vi "Chaser_Mk2.vi"   [LabVIEW 2015]
uses:
  <vilib>/Aledyne-TSXperts/Arduino Compatible Compiler for LabVIEW/Code Generator/Arduino APIs/RGB LED Strip/RGB Strip Mode.ctl
  <vilib>/Aledyne-TSXperts/Arduino Compatible Compiler for LabVIEW/Code Generator/Arduino APIs/Serial/Serial Settings.ctl
  <vilib>/Aledyne-TSXperts/Arduino Compatible Compiler for LabVIEW/Arduino Compatible Compiler for LabVIEW.lvlib
types:
  T1 = typedef "Arduino Compatible Compiler for LabVIEW.lvlib/Serial Settings.ctl" = u16
  T2 = typedef "Arduino Compatible Compiler for LabVIEW.lvlib/RGB Strip Mode.ctl" = u16
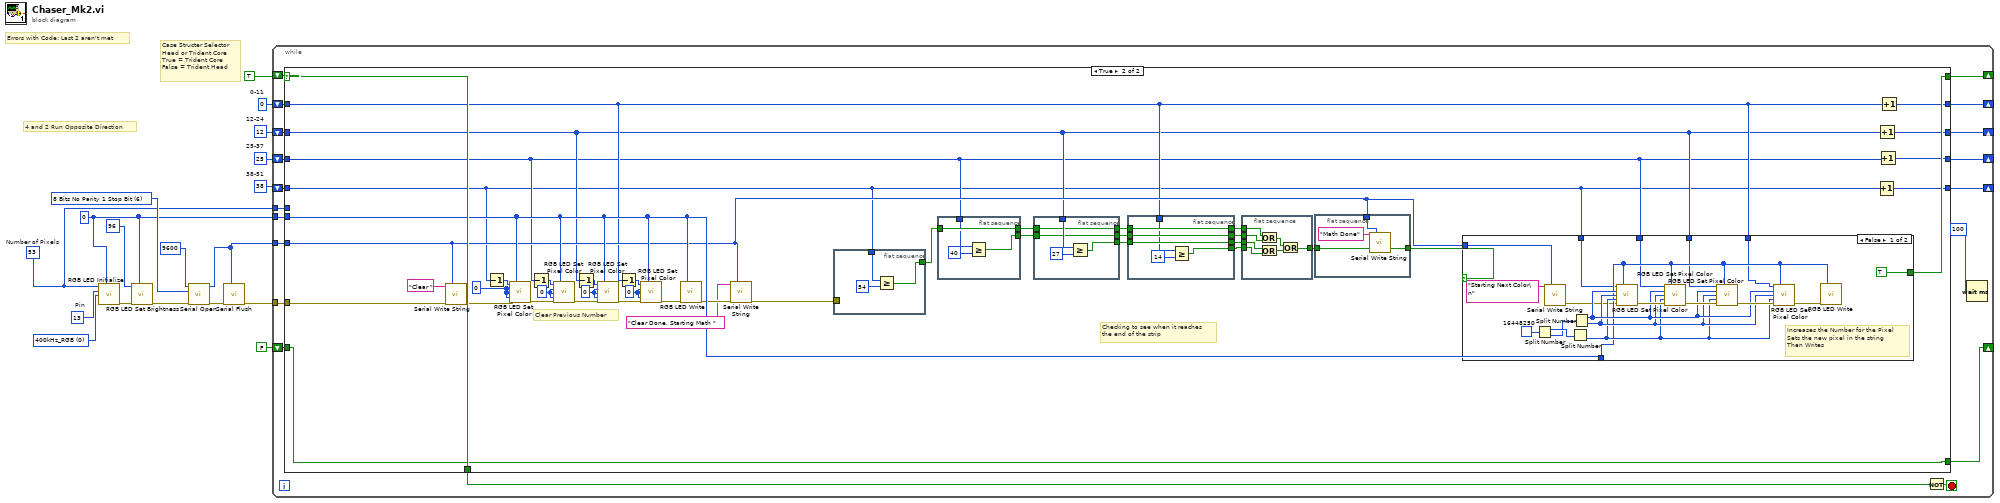
[diagram p0: block diagram]
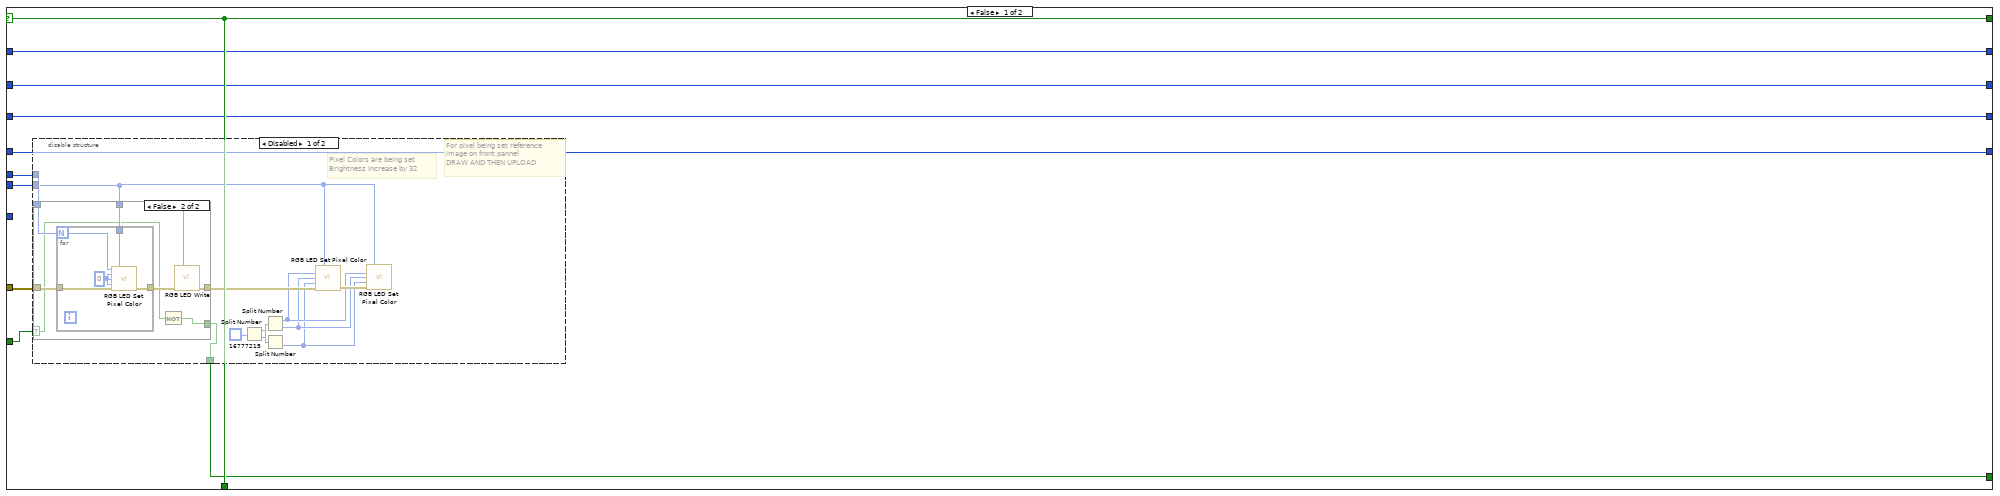
[diagram p2: hidden frame]
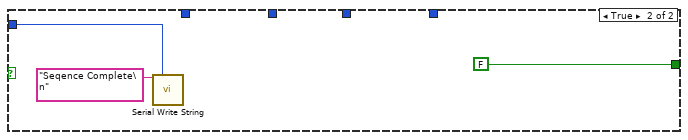
[diagram p5: hidden frame]
diagram:
  w5 = u16 38  # 38-51
  w6 = u16 25  # 25-37
  w7 = u16 12  # 12-24
  w8 = u16 0  # 0-11
  w13 = T1 6 items=["5 Bits No Parity 1 Stop Bit"=0, "6 Bits No Parity 1 Stop Bit"=2, "7 Bits No Parity 1 Stop Bit"=4, "8 Bits No Parity 1 Stop Bit"=6, "5 Bits No Parity 2 Stop Bits"=8, "6 Bits No Parity 2 Stop Bits"=10, "7 Bits No Parity 2 Stop Bits"=12, "8 Bits No Parity 2 Stop Bits"=14, "5 Bits Even Parity 1 Stop Bits"=32, "6 Bits Even Parity 1 Stop Bits"=34, "7 Bits Even Parity 1 Stop Bits"=36, "8 Bits Even Parity 1 Stop Bits"=38, "5 Bits Even Parity 2 Stop Bits"=40, "6 Bits Even Parity 2 Stop Bits"=42, "7 Bits Even Parity 2 Stop Bits"=44, "8 Bits Even Parity 2 Stop Bits"=46, "5 Bits Odd Parity 1 Stop Bits"=48, "6 Bits Odd Parity 1 Stop Bits"=50, "7 Bits Odd Parity 1 Stop Bits"=52, "8 Bits Odd Parity 1 Stop Bits"=54, "5 Bits Odd Parity 2 Stop Bits"=56, "6 Bits Odd Parity 2 Stop Bits"=58, "7 Bits Odd Parity 2 Stop Bits"=60, "8 Bits Odd Parity 2 Stop Bits"=62] ("Serial Settings")
  w17 = T2 0 items=["400kHz_RGB"=0, "400kHz_GRB"=1, "400kHz_BRG"=4, "800kHz_RGB"=2, "800kHz_GRB"=3, "400kHz_BRG"=6] ("Mode")
  w18 = u8 13  # Pin
  w2 = u8 53  # Number of Pixels
  w4 = u8 0 ("Instance")
  # "Errors with Code: Last 2 aren't met"
  # "4 and 2 Run Opposite Direction"
  # "Case Structer Selector\nHead or Trident Core\nTrue = Trident Core\nFalse = Trident Head"
  n1 = call <vilib>:"RGB LED Initialize.vi"("Number of Pixels"=w2, "Instance"=w4, "Pin"=w18, "Mode"=w17) -> ("error out"=w16:errorcluster)  [unwired: 11 in]
  n2 = call <vilib>:"RGB LED Set Brightness.vi"("Brightness"=u8 96, "Instance"=w4, "error in (no error)"=w16) -> ("error out"=w14:errorcluster)  [unwired: 12 in]
  n3 = call <vilib>:"Serial Open.vi"("Speed"=u32 9600, "Serial Settings"=w13, "error in (no error)"=w14) -> ("Instance"=w3:u8, "error out"=w11:errorcluster)  [unwired: 11 in]
  n4 = call <vilib>:"Serial Flush.vi"("Instance"=w3, "error in (no error)"=w11) -> ("error out"=w10:errorcluster)  [unwired: 13 in]
  n5 = while {
    tunnel: w10 -> [w29]
    shift-right: [w36] -> _
    shift-left: TRUE -> [w37]
    shift-right: [w27] -> _
    shift-left: w8 -> [w33]
    shift-right: [w26] -> _
    shift-left: w7 -> [w32]
    shift-right: [w25] -> _
    shift-left: w6 -> [w31]
    shift-right: [w24] -> _
    shift-left: w5 -> [w30]
    tunnel: w4 -> [w28]
    tunnel: w3 -> [w23]
    tunnel: w2 -> [w21]
    shift-right: [w19] -> _
    shift-left: FALSE -> [w20]
    stop <- w35 stop-if-true
    n6 = case shown="True" w37 {
      selector: w37 -> [w47 w98]
      tunnel: [w47 w97] -> w36
      tunnel: [w47 w98] -> w34
      tunnel: w33 -> [w46 w83]
      tunnel: w32 -> [w45 w81]
      tunnel: w31 -> [w44 w78]
      tunnel: w30 -> [w43 w76]
      tunnel: w29 -> [w41 w88]
      tunnel: w28 -> [w38 w96]
      tunnel: [w46 w82] -> w27
      tunnel: [w45 w80] -> w26
      tunnel: [w44 w79] -> w25
      tunnel: [w43 w77] -> w24
      tunnel: w23 -> [_ w89]
      tunnel: w21 -> [w42 _]
      tunnel: w20 -> [w40 w75]
      tunnel: [w39 w75] -> w19
      frame False {
        n7 = disable-structure shown="Disabled" {
          disable-tunnel: w42 -> [w60 _]
          disable-tunnel: w41 -> [w59 _]
          disable-tunnel: w40 -> [w58 _]
          disable-tunnel: [w57 _] -> w39
          disable-tunnel: w38 -> [w48 _]
          frame Disabled {
            # "For pixel being set reference\nimage on front pannel\nDRAW AND THEN UPLOAD"
            # "Pixel Colors are being set\nBrightness Increase by 32"
            n8 = case shown="False" w58 {
              selector: w58 -> [w61 w64]
              tunnel: w60 -> [_ w69]
              tunnel: w59 -> [w62 w68]
              tunnel: w48 -> [_ w66]
              tunnel: [w62 w65] -> w56
              tunnel: [w61 w63] -> w57
              frame True {
              }
              frame False {
                n9 = for {
                  N: w69 -> [w73]
                  tunnel: w68 -> [w74]
                  tunnel: w66 -> [w71]
                  tunnel: [w70] -> w67
                  w72 = u8 0 ("Green")
                  n10 = call <vilib>:"RGB LED Set Pixel Color.vi"("Pixel"=w73, "Instance"=w71, "Red"=w72, "Green"=w72, "Blue"=w72, "error in (no error)"=w74) -> ("error out"=w70:errorcluster)  [unwired: 9 in]
                }
                n11 = Not(x=w64) -> (.not. x?=w63:bool)
                n12 = call <vilib>:"RGB LED Write.vi"("Instance"=w66, "error in (no error)"=w67) -> ("error out"=w65:errorcluster)  [unwired: 13 in]
              }
            }
            n13 = Split Number(x=u32 16777215) -> (hi(x)=w54:u16, lo(x)=w53:u16)
            n14 = Split Number(x=w53) -> (hi(x)=w51:u8, lo(x)=w50:u8)
            n15 = Split Number(x=w54) -> (lo(x)=w49:u8)  [unwired: 1 out]
            n16 = call <vilib>:"RGB LED Set Pixel Color.vi"("Instance"=w48, "Red"=w51, "Green"=w50, "Blue"=w49, "error in (no error)"=w56) -> ("error out"=w52:errorcluster)  [unwired: 10 in]
            n17 = call <vilib>:"RGB LED Set Pixel Color.vi"("Instance"=w48, "Red"=w51, "Green"=w50, "Blue"=w49, "error in (no error)"=w52) -> ()  [unwired: 10 in, 1 out]
          }
          frame Enabled {
          }
        }
      }
      frame True {
        w112 = u8 0 ("Green")
        w113 = u8 0 ("Green")
        w115 = u8 0 ("Green")
        w116 = u8 0 ("Green")
        # "Checking to see when it reaches\nthe end of the strip"
        # "Clear Previous Number"
        n18 = call <vilib>:"Serial Write String.vi"("String"="Clear ", "Instance"=w89, "error in (no error)"=w88) -> ("error out"=w93:errorcluster)  [unwired: 12 in]
        n19 = Decrement(x=w76) -> (x-1=w87:u16)
        n20 = call <vilib>:"RGB LED Set Pixel Color.vi"("Pixel"=w87, "Instance"=w96, "Red"=w116, "Green"=w116, "Blue"=w116, "error in (no error)"=w93) -> ("error out"=w114:errorcluster)  [unwired: 9 in]
        n21 = Decrement(x=w78) -> (x-1=w86:u16)
        n22 = call <vilib>:"RGB LED Set Pixel Color.vi"("Pixel"=w86, "Instance"=w96, "Red"=w115, "Green"=w115, "Blue"=w115, "error in (no error)"=w114) -> ("error out"=w110:errorcluster)  [unwired: 9 in]
        n23 = Decrement(x=w81) -> (x-1=w85:u16)
        n24 = call <vilib>:"RGB LED Set Pixel Color.vi"("Pixel"=w85, "Instance"=w96, "Red"=w113, "Green"=w113, "Blue"=w113, "error in (no error)"=w110) -> ("error out"=w111:errorcluster)  [unwired: 9 in]
        n25 = Decrement(x=w83) -> (x-1=w84:u16)
        n26 = call <vilib>:"RGB LED Set Pixel Color.vi"("Pixel"=w84, "Instance"=w96, "Red"=w112, "Green"=w112, "Blue"=w112, "error in (no error)"=w111) -> ("error out"=w109:errorcluster)  [unwired: 9 in]
        n27 = call <vilib>:"RGB LED Write.vi"("Instance"=w96, "error in (no error)"=w109) -> ("error out"=w95:errorcluster)  [unwired: 13 in]
        n28 = call <vilib>:"Serial Write String.vi"("String"="Clear Done. Starting Math ", "Instance"=w89, "error in (no error)"=w95) -> ()  [unwired: 12 in, 1 out]
        n29 = flat-sequence {
          tunnel: w95 -> [_]
          tunnel: w76 -> [w164]
          tunnel: [w165] -> w108
          frame #0 {
            n30 = Greater Or Equal?(x=w164, y=u16 54) -> (x >= y?=w165:bool)
          }
        }
        n31 = flat-sequence {
          tunnel: w108 -> [w163]
          tunnel: [w163] -> w107
          tunnel: w78 -> [w162]
          tunnel: [w161] -> w106
          frame #0 {
            n32 = Greater Or Equal?(x=w162, y=u16 40) -> (x >= y?=w161:bool)
          }
        }
        n33 = flat-sequence {
          tunnel: w107 -> [w158]
          tunnel: w106 -> [w157]
          tunnel: w81 -> [w159]
          tunnel: [w158] -> w103
          tunnel: [w157] -> w104
          tunnel: [w155] -> w105
          frame #0 {
            n34 = Greater Or Equal?(x=w159, y=u16 27) -> (x >= y?=w155:bool)
          }
        }
        n35 = flat-sequence {
          tunnel: w105 -> [w152]
          tunnel: w104 -> [w153]
          tunnel: w103 -> [w154]
          tunnel: w83 -> [w151]
          tunnel: [w154] -> w102
          tunnel: [w153] -> w101
          tunnel: [w152] -> w100
          tunnel: [w149] -> w99
          frame #0 {
            n36 = Greater Or Equal?(x=w151, y=u16 14) -> (x >= y?=w149:bool)
          }
        }
        n37 = flat-sequence {
          tunnel: w102 -> [w146]
          tunnel: w101 -> [w145]
          tunnel: w100 -> [w144]
          tunnel: w99 -> [w143]
          tunnel: [w142] -> w91
          frame #0 {
            n38 = Or(x=w146, y=w145) -> (x .or. y?=w147:bool)
            n39 = Or(x=w144, y=w143) -> (x .or. y?=w148:bool)
            n40 = Or(x=w147, y=w148) -> (x .or. y?=w142:bool)
          }
        }
        n41 = flat-sequence {
          tunnel: [w119] -> w90
          tunnel: w91 -> [w119]
          tunnel: w89 -> [w117]
          frame #0 {
            n42 = call <vilib>:"Serial Write String.vi"("String"="Math Done", "Instance"=w117) -> ()  [unwired: 13 in, 1 out]
          }
        }
        n43 = case shown="False" w90 {
          tunnel: [TRUE FALSE] -> w97
          tunnel: w76 -> [w123 _]
          tunnel: w96 -> [w127 _]
          tunnel: w78 -> [w122 _]
          tunnel: w81 -> [w121 _]
          tunnel: w83 -> [w120 _]
          tunnel: w89 -> [w124 w139]
          frame False {
            # "Increases the Number for the Pixel\nSets the new pixel in the string\nThen Writes"
            n44 = Split Number(x=u32 16448250) -> (hi(x)=w136:u16, lo(x)=w135:u16)
            n45 = call <vilib>:"Serial Write String.vi"("String"="Starting Next Color\n", "Instance"=w124) -> ("error out"=w126:errorcluster)  [unwired: 13 in]
            n46 = Split Number(x=w136) -> (lo(x)=w129:u8)  [unwired: 1 out]
            n47 = Split Number(x=w135) -> (hi(x)=w131:u8, lo(x)=w130:u8)
            n48 = call <vilib>:"RGB LED Set Pixel Color.vi"("Pixel"=w123, "Instance"=w127, "Red"=w131, "Green"=w130, "Blue"=w129, "error in (no error)"=w126) -> ("error out"=w134:errorcluster)  [unwired: 9 in]
            n49 = call <vilib>:"RGB LED Set Pixel Color.vi"("Pixel"=w122, "Instance"=w127, "Red"=w131, "Green"=w130, "Blue"=w129, "error in (no error)"=w134) -> ("error out"=w133:errorcluster)  [unwired: 9 in]
            n50 = call <vilib>:"RGB LED Set Pixel Color.vi"("Pixel"=w121, "Instance"=w127, "Red"=w131, "Green"=w130, "Blue"=w129, "error in (no error)"=w133) -> ("error out"=w132:errorcluster)  [unwired: 9 in]
            n51 = call <vilib>:"RGB LED Set Pixel Color.vi"("Pixel"=w120, "Instance"=w127, "Red"=w131, "Green"=w130, "Blue"=w129, "error in (no error)"=w132) -> ("error out"=w128:errorcluster)  [unwired: 9 in]
            n52 = call <vilib>:"RGB LED Write.vi"("Instance"=w127, "error in (no error)"=w128) -> ()  [unwired: 13 in, 1 out]
          }
          frame True {
            n53 = call <vilib>:"Serial Write String.vi"("String"="Seqence Complete\n", "Instance"=w139) -> ()  [unwired: 13 in, 1 out]
          }
        }
        n54 = Increment(x=w76) -> (x+1=w77:u16)
        n55 = Increment(x=w81) -> (x+1=w80:u16)
        n56 = Increment(x=w78) -> (x+1=w79:u16)
        n57 = Increment(x=w83) -> (x+1=w82:u16)
      }
    }
    n58 = Not(x=w34) -> (.not. x?=w35:bool)
    n59 = Wait (ms)(milliseconds to wait=u32 100) -> ()  [unwired: 1 out]
  }
